vi "send_TLC.vi"(8 "error in (no error)":errorcluster, 11 "GenericToplevelComponent in":refnum<class "GenericToplevelComponent.lvclass">) -> (0 "error out":errorcluster, 3 "GenericToplevelComponent out":refnum<class "GenericToplevelComponent.lvclass">)   [LabVIEW 2010, in "GenericToplevelComponent.lvclass"]
uses:
  GenericToplevelComponent.lvclass
  class_data.vi
  GenericComponent/GenericComponent/GenericComponent.lvclass
panel:
  out "# elements in queue":i32
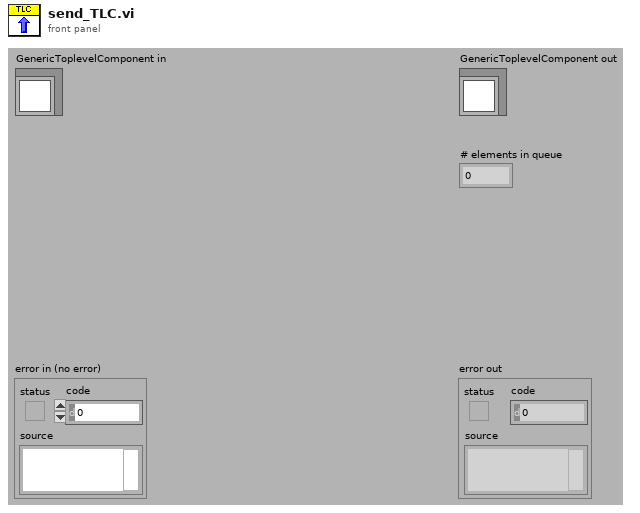
[diagram p1: front panel]
types:
  T1 = typedef "GenericToplevelComponent.lvclass/common_trigger_enum.ctl" = enum16{"NULL", "initialise", "terminate", "fetch command", "fetch data", "attach observer", "register as observer", "detach observer", "acknowledge", "start", "stop", "sweep started", "sweep finished", "experiment started", "experiment stopped"}
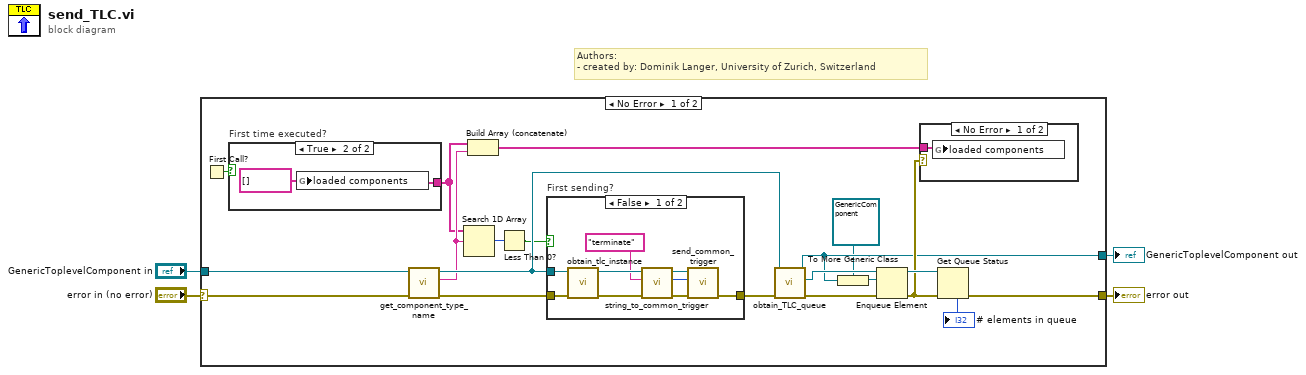
[diagram p0: block diagram]
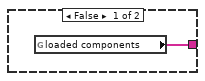
[diagram p2: hidden frame]
diagram:
  # "Authors: \n- created by: Dominik Langer, University of Zurich, Switzerland"
  n1 = case shown="No Error" "error in (no error)" {
    selector: "error in (no error)" -> [w19 w39]
    tunnel: [w21 w39] -> w3
    tunnel: [w7 w38] -> w1
    tunnel: "GenericToplevelComponent in" -> [w17 w38]
    frame No Error {
      n2 = First Call?() -> (First Call?: T/F=w9:bool)
      n3 = case "First time executed?" shown="True" w9 {
        tunnel: [w25 w26] -> w8
        frame False {
          n4 = global read "class_data.vi" "loaded components"() -> (w25:string[])
        }
        frame True {
          w26 = string[] [] ("loaded components")
          n5 = global write "class_data.vi" "loaded components"(w26) -> ()
        }
      }
      n6 = call-dynamic "get_component_type_name.vi"("error in (no error)"=w19, "GenericPlugin in"=w17) -> ("error out"=w18:errorcluster, "component type"=w12:string, "GenericPlugin out"=w16:refnum<class "GenericToplevelComponent.lvclass">)  [unwired: 7 in]
      n7 = Search 1D Array(1D array=w8, element=w12) -> (index of element=w15:i32)  [unwired: 1 in]
      n8 = Build Array (concatenate)(w8, w12) -> (w11:string[])
      n9 = Less Than 0?(x=w15) -> (x < 0?=w14:bool)
      n10 = case "First sending?" shown="False" w14 {
        tunnel: w18 -> [w35 w37]
        tunnel: [w36 w37] -> w20
        tunnel: w16 -> [w34 _]
        frame False {
          n11 = call-dynamic "obtain_tlc_instance.vi"("error in (no error)"=w35, "GenericToplevelComponent in"=w34) -> ("error out"=w33:errorcluster, "GenericToplevelComponent out"=w31:refnum<class "GenericToplevelComponent.lvclass">)  [unwired: 8 in]
          n12 = call-dynamic "string_to_common_trigger.vi"("error in (no error)"=w33, "trigger string"="terminate", "GenericToplevelComponent in"=w31) -> ("error out"=w32:errorcluster, "trigger"=w29:T1, "GenericToplevelComponent out"=w30:refnum<class "GenericToplevelComponent.lvclass">)  [unwired: 6 in]
          n13 = call-dynamic "send_common_trigger.vi"("error in (no error)"=w32, "trigger"=w29, "GenericToplevelComponent in"=w30) -> ("error out"=w36:errorcluster)  [unwired: 6 in, 2 out]
        }
        frame True {
        }
      }
      n14 = call-dynamic "obtain_TLC_queue.vi"("error in (no error)"=w20, "GenericToplevelComponent in"=w16) -> ("error out"=w23:errorcluster, "TLC queue"=w24:refnum<queue>, "GenericToplevelComponent out"=w7:refnum<class "GenericToplevelComponent.lvclass">)  [unwired: 7 in]
      n15 = To More Generic Class(target class=refnum<class "GenericComponent.lvclass"> refnum ("GenericComponent.lvclass"), reference=w7) -> (generic class reference=w6:refnum<class "GenericComponent.lvclass">)
      n16 = Enqueue Element(queue=w24, element=w6, error in (no error)=w23) -> (queue out=w22:refnum<queue>, error out=w13:errorcluster)  [unwired: 1 in, 1 out]
      n17 = case shown="No Error" w13 {
        tunnel: w11 -> [w27 _]
        frame No Error {
          n18 = global write "class_data.vi" "loaded components"(w27) -> ()
        }
        frame Error {
        }
      }
      n19 = Get Queue Status(queue=w22, error in (no error)=w13) -> (error out=w21:errorcluster, # elements in queue=→"# elements in queue":i32)  [unwired: 1 in, 6 out]
    }
    frame Error {
    }
  }
  "error out" <- w3
  "GenericToplevelComponent out" <- w1
